vi "Mod6DIOaus.vi"   [LabVIEW 2017]
uses:
  <vilib>/rvi/eio/common/nirviEmuTemplateMethod_errors.vi
  <vilib>/eio/EIONode/EIONode.xnode
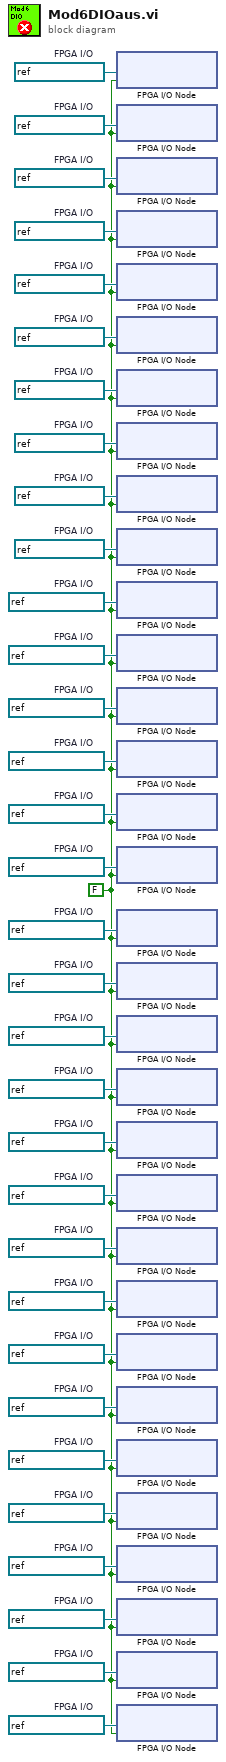
[diagram p0: block diagram]
diagram:
  w1 = FALSE ("I/O Item")
  w2 = refnum<k21> "Mod6/DIO31"  # FPGA I/O
  w3 = refnum<k21> "Mod6/DIO30"  # FPGA I/O
  w4 = refnum<k21> "Mod6/DIO29"  # FPGA I/O
  w5 = refnum<k21> "Mod6/DIO28"  # FPGA I/O
  w6 = refnum<k21> "Mod6/DIO27"  # FPGA I/O
  w7 = refnum<k21> "Mod6/DIO26"  # FPGA I/O
  w8 = refnum<k21> "Mod6/DIO25"  # FPGA I/O
  w9 = refnum<k21> "Mod6/DIO24"  # FPGA I/O
  w10 = refnum<k21> "Mod6/DIO23"  # FPGA I/O
  w11 = refnum<k21> "Mod6/DIO22"  # FPGA I/O
  w12 = refnum<k21> "Mod6/DIO21"  # FPGA I/O
  w13 = refnum<k21> "Mod6/DIO20"  # FPGA I/O
  w14 = refnum<k21> "Mod6/DIO19"  # FPGA I/O
  w15 = refnum<k21> "Mod6/DIO18"  # FPGA I/O
  w16 = refnum<k21> "Mod6/DIO17"  # FPGA I/O
  w17 = refnum<k21> "Mod6/DIO16"  # FPGA I/O
  w18 = refnum<k21> "Mod6/DIO15"  # FPGA I/O
  w19 = refnum<k21> "Mod6/DIO14"  # FPGA I/O
  w20 = refnum<k21> "Mod6/DIO13"  # FPGA I/O
  w21 = refnum<k21> "Mod6/DIO12"  # FPGA I/O
  w22 = refnum<k21> "Mod6/DIO11"  # FPGA I/O
  w23 = refnum<k21> "Mod6/DIO10"  # FPGA I/O
  w24 = refnum<k21> "Mod6/DIO9"  # FPGA I/O
  w25 = refnum<k21> "Mod6/DIO8"  # FPGA I/O
  w26 = refnum<k21> "Mod6/DIO7"  # FPGA I/O
  w27 = refnum<k21> "Mod6/DIO6"  # FPGA I/O
  w28 = refnum<k21> "Mod6/DIO5"  # FPGA I/O
  w29 = refnum<k21> "Mod6/DIO4"  # FPGA I/O
  w30 = refnum<k21> "Mod6/DIO3"  # FPGA I/O
  w31 = refnum<k21> "Mod6/DIO2"  # FPGA I/O
  w32 = refnum<k21> "Mod6/DIO1"  # FPGA I/O
  w33 = refnum<k21> "Mod6/DIO0"  # FPGA I/O
  n1 = xnode "FPGA I/O Node"("I/O-Objekt"=w1, "FPGA-I/O (Eingang)"=w33) -> ()  [unwired: 1 out]
  n2 = xnode "FPGA I/O Node"("I/O-Objekt"=w1, "FPGA-I/O (Eingang)"=w32) -> ()  [unwired: 1 out]
  n3 = xnode "FPGA I/O Node"("I/O-Objekt"=w1, "FPGA-I/O (Eingang)"=w31) -> ()  [unwired: 1 out]
  n4 = xnode "FPGA I/O Node"("I/O-Objekt"=w1, "FPGA-I/O (Eingang)"=w30) -> ()  [unwired: 1 out]
  n5 = xnode "FPGA I/O Node"("I/O-Objekt"=w1, "FPGA-I/O (Eingang)"=w29) -> ()  [unwired: 1 out]
  n6 = xnode "FPGA I/O Node"("I/O-Objekt"=w1, "FPGA-I/O (Eingang)"=w28) -> ()  [unwired: 1 out]
  n7 = xnode "FPGA I/O Node"("I/O-Objekt"=w1, "FPGA-I/O (Eingang)"=w27) -> ()  [unwired: 1 out]
  n8 = xnode "FPGA I/O Node"("I/O-Objekt"=w1, "FPGA-I/O (Eingang)"=w26) -> ()  [unwired: 1 out]
  n9 = xnode "FPGA I/O Node"("I/O-Objekt"=w1, "FPGA-I/O (Eingang)"=w25) -> ()  [unwired: 1 out]
  n10 = xnode "FPGA I/O Node"("I/O-Objekt"=w1, "FPGA-I/O (Eingang)"=w24) -> ()  [unwired: 1 out]
  n11 = xnode "FPGA I/O Node"("I/O-Objekt"=w1, "FPGA-I/O (Eingang)"=w23) -> ()  [unwired: 1 out]
  n12 = xnode "FPGA I/O Node"("I/O-Objekt"=w1, "FPGA-I/O (Eingang)"=w22) -> ()  [unwired: 1 out]
  n13 = xnode "FPGA I/O Node"("I/O-Objekt"=w1, "FPGA-I/O (Eingang)"=w21) -> ()  [unwired: 1 out]
  n14 = xnode "FPGA I/O Node"("I/O-Objekt"=w1, "FPGA-I/O (Eingang)"=w20) -> ()  [unwired: 1 out]
  n15 = xnode "FPGA I/O Node"("I/O-Objekt"=w1, "FPGA-I/O (Eingang)"=w19) -> ()  [unwired: 1 out]
  n16 = xnode "FPGA I/O Node"("I/O-Objekt"=w1, "FPGA-I/O (Eingang)"=w18) -> ()  [unwired: 1 out]
  n17 = xnode "FPGA I/O Node"("I/O-Objekt"=w1, "FPGA-I/O (Eingang)"=w17) -> ()  [unwired: 1 out]
  n18 = xnode "FPGA I/O Node"("I/O-Objekt"=w1, "FPGA-I/O (Eingang)"=w16) -> ()  [unwired: 1 out]
  n19 = xnode "FPGA I/O Node"("I/O-Objekt"=w1, "FPGA-I/O (Eingang)"=w15) -> ()  [unwired: 1 out]
  n20 = xnode "FPGA I/O Node"("I/O-Objekt"=w1, "FPGA-I/O (Eingang)"=w14) -> ()  [unwired: 1 out]
  n21 = xnode "FPGA I/O Node"("I/O-Objekt"=w1, "FPGA-I/O (Eingang)"=w13) -> ()  [unwired: 1 out]
  n22 = xnode "FPGA I/O Node"("I/O-Objekt"=w1, "FPGA-I/O (Eingang)"=w12) -> ()  [unwired: 1 out]
  n23 = xnode "FPGA I/O Node"("I/O-Objekt"=w1, "FPGA-I/O (Eingang)"=w11) -> ()  [unwired: 1 out]
  n24 = xnode "FPGA I/O Node"("I/O-Objekt"=w1, "FPGA-I/O (Eingang)"=w10) -> ()  [unwired: 1 out]
  n25 = xnode "FPGA I/O Node"("I/O-Objekt"=w1, "FPGA-I/O (Eingang)"=w9) -> ()  [unwired: 1 out]
  n26 = xnode "FPGA I/O Node"("I/O-Objekt"=w1, "FPGA-I/O (Eingang)"=w8) -> ()  [unwired: 1 out]
  n27 = xnode "FPGA I/O Node"("I/O-Objekt"=w1, "FPGA-I/O (Eingang)"=w7) -> ()  [unwired: 1 out]
  n28 = xnode "FPGA I/O Node"("I/O-Objekt"=w1, "FPGA-I/O (Eingang)"=w6) -> ()  [unwired: 1 out]
  n29 = xnode "FPGA I/O Node"("I/O-Objekt"=w1, "FPGA-I/O (Eingang)"=w5) -> ()  [unwired: 1 out]
  n30 = xnode "FPGA I/O Node"("I/O-Objekt"=w1, "FPGA-I/O (Eingang)"=w4) -> ()  [unwired: 1 out]
  n31 = xnode "FPGA I/O Node"("I/O-Objekt"=w1, "FPGA-I/O (Eingang)"=w3) -> ()  [unwired: 1 out]
  n32 = xnode "FPGA I/O Node"("I/O-Objekt"=w1, "FPGA-I/O (Eingang)"=w2) -> ()  [unwired: 1 out]
